vi "求组合（化简公式）.vi"(1 "k":u32=100, 2 "n":u32=100) -> (0 "C(n,k)":dbl)   [LabVIEW 2012]
doc: "功能：\n\n利用化简组合公式求组合。\n\n公式：\n\nC(n,k)=n!/(k!*(n-k)!\n\n根据阶乘的定义，n!可以被k!或者（n-k）的阶乘约分，因此可以选择k和n-k中较大的进行约分，极大地减少了循环次数，避免了阶乘溢出的问题。\n\n\nCSXCS_366创建"
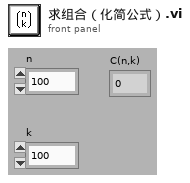
[diagram p1: front panel]
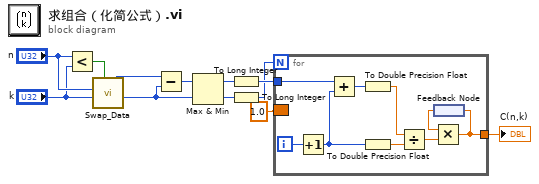
[diagram p0: block diagram]
diagram:
  n1 = Less?(x="n", y="k") -> (x < y?=w8:bool)
  n2 = call-poly "Swap_Data.vi"("Swap(T)"=w8, "b"="k", "a"="n") -> ("b"=w4:u32, "a"=w7:u32)  [unwired: 4 in]
  n3 = Subtract(x=w7, y=w4) -> (x-y=w12:u32)
  n4 = Max & Min(x=w12, y=w4) -> (max(x,y)=w10:u32, min(x,y)=w11:u32)
  n5 = To Long Integer(number=w10) -> (32bit integer=w2:i32)
  n6 = To Long Integer(number=w11) -> (32bit integer=w1:i32)
  n7 = for {
    N: w1 -> [_]
    tunnel: w2 -> [w21]
    tunnel: [w14] -> w9
    border: 1.0 ("C(n,k)") -> [_]
    i -> [w20]
    n8 = Increment(x=w20) -> (x+1=w18:i32)
    n9 = Add(x=w21, y=w18) -> (x+y=w19:i32)
    n10 = To Double Precision Float(number=w19) -> (double precision float=w16:dbl)
    n11 = To Double Precision Float(number=w18) -> (double precision float=w15:dbl)
    n12 = Divide(x=w16, y=w15) -> (x/y=w17:dbl)
    n13 = feedback #1() -> (w13:dbl)
    n14 = Multiply(x=w13, y=w17) -> (x*y=w14:dbl)
    n15 = feedback-in #1(w14) -> ()
  }
  "C(n,k)" <- w9
